vi "Calculate Gradients.vi"(9 "Bottom":T2, 10 "Middle":T2, 11 "Top":T2) -> (1 "Middle --> Bottom":T1, 2 "Line Top --> Middle":T1, 3 "Line Top --> Bottom":T1)   [LabVIEW 2022 SP3, in "Raster.lvlib"]
uses:
  Raster.lvlib
  Point 2D.ctl
  Line Parameters.ctl
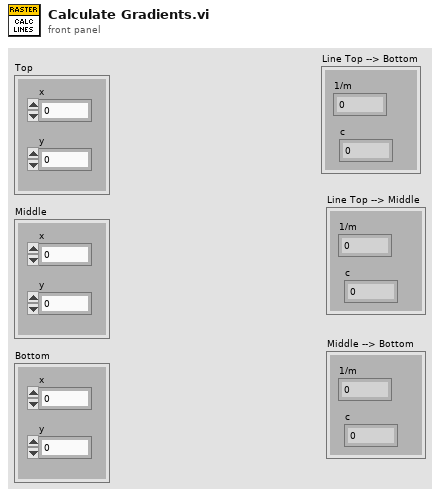
[diagram p1: front panel]
types:
  T1 = typedef "Raster.lvlib/Line Parameters.ctl" = cluster{"1/m":dbl, "c":dbl}
  T2 = typedef "Raster.lvlib/Point 2D.ctl" = cluster{"x":i32, "y":i32}
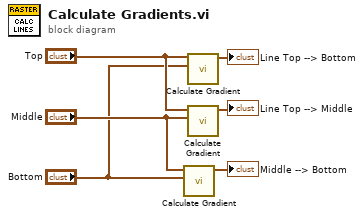
[diagram p0: block diagram]
diagram:
  n1 = call "Calculate Gradient.vi"("P2"="Bottom", "P1"="Middle") -> ("Line Parameters"=→"Middle --> Bottom":T1)  [unwired: 9 in]
  n2 = call "Calculate Gradient.vi"("P2"="Bottom", "P1"="Top") -> ("Line Parameters"=→"Line Top --> Bottom":T1)  [unwired: 9 in]
  n3 = call "Calculate Gradient.vi"("P2"="Middle", "P1"="Top") -> ("Line Parameters"=→"Line Top --> Middle":T1)  [unwired: 9 in]
